vi "Date Server Queue.vi"(2 "新值":T1, 3 "set queue? (F: de-queue)":bool caption="设置队列？（F: 取消队列）") -> (0 "值":T1, 1 "valid?":bool caption="有效？")   [LabVIEW 2016]
doc: "保存至Data Server.vi的每个TCP连接的功能全局变量将生成引用句柄数组。\n\n<B>注：</B>用于Data & Time Server.vi的子VI必须位于TCP库中。"
panel:
  in  "empty":refnum<k5> caption="空"
  # "注： 与\"Multiple Connections - Server.vi\"一起使用"
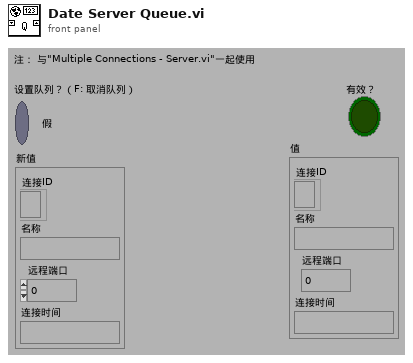
[diagram p1: front panel]
types:
  T1 = cluster{"连接ID":refnum<k5>, "名称":string, "远程端口":u16, "连接时间":string}
  T2 = cluster{"连接ID":refnum<k5>, "名称":string, "远程端口":u16, "连接时间":string}[]
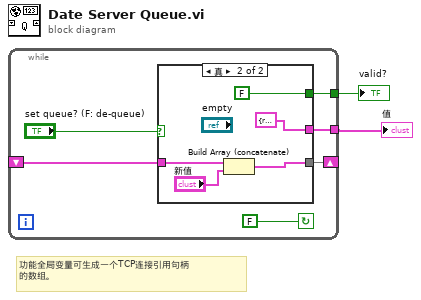
[diagram p0: block diagram]
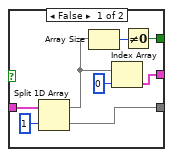
[diagram p2: hidden frame]
diagram:
  # "功能全局变量可生成一个TCP连接引用句柄\n的数组。"
  n1 = while {
    tunnel: [w4] -> w2
    tunnel: [w5] -> w1
    shift-left: _ -> [w7]
    shift-right: [w8] -> _
    stop <- FALSE continue-if-true
    n2 = case shown="真" "set queue? (F: de-queue)" {
      tunnel: [w14 w21] -> w8
      tunnel: w7 -> [w16 w20]
      tunnel: [w11 T1 {"连接ID"=refnum, "名称"="", "远程端口"=0, "连接时间"=""}] -> w5
      tunnel: [w9 FALSE] -> w4
      frame False {
        n3 = Split 1D Array(array=w16, index=1) -> (first subarray=w12:T2, second subarray=w14:T2)
        n4 = Array Size(array=w12) -> (size(s)=w10:i32)
        n5 = Index Array(array=w12, index=0) -> (element=w11:T1)
        n6 = Not Equal To 0?(x=w10) -> (x != 0?=w9:bool)
      }
      frame True {
        n7 = Build Array (concatenate)(w20, "新值") -> (w21:T2)
      }
    }
  }
  "valid?" <- w2
  "值" <- w1
